vi "GetWindowICCProfile.vi"(8 "No Error":errorcluster, 11 "Window [SDL_Window *]":i64 format="%.0x") -> (0 "Error Out":errorcluster, 3 "ICC Profile Data":u8[](array[numeric]))   [LabVIEW 2026, in "SDL3.lvlib" / "Video.lvlib"]
doc: "<B>Summary</B>\nGet the raw ICC profile data for the screen the window is currently on."
uses:
  Video.lvlib
  <vilib>/Utility/error.llb/Error Cluster From Error Code.vi
  Stdinc/Stdinc.lvlib
  Error/Error.lvlib
  Lib/SDL3.dll
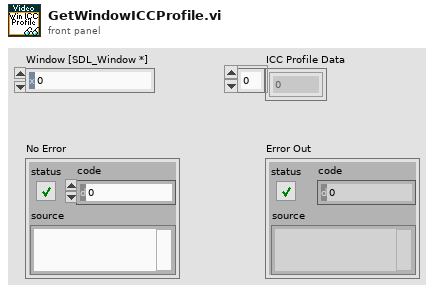
[diagram p1: front panel]
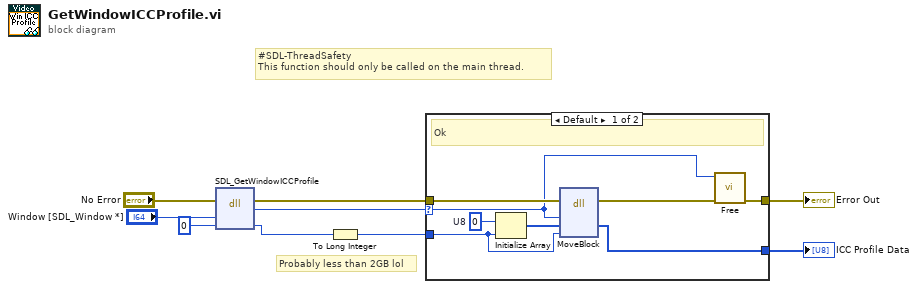
[diagram p0: block diagram]
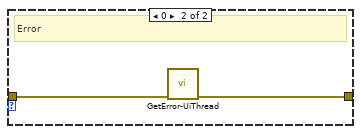
[diagram p2: hidden frame]
diagram:
  # "#SDL-ThreadSafety\nThis function should only be called on the main thread."
  # "Probably less than 2GB lol"
  n1 = dll-call lib="C:/Users/saukko/Dev/LV-SDL3/Sources/SDL3/Lib/SDL3.*" fn="SDL_GetWindowICCProfile"(error in="No Error", "window"="Window [SDL_Window *]", "size"=u64 0) -> (error out=w7:errorcluster, "return type"=w6:i64, "size"=w5:u64)  [unwired: 3 in, 1 out]
  n2 = To Long Integer(number=w5) -> (32bit integer=w2:i32)
  n3 = case shown="Default" w6 {
    selector: w6 -> [w12 _]
    tunnel: w7 -> [w17 w19]
    tunnel: [w13 w18] -> w8
    tunnel: w2 -> [w10 _]
    tunnel: [w14 _] -> w1
    frame Default {
      w11 = u8 0  # U8
      # "Ok"
      n4 = Initialize Array(w11, w10) -> (w15:u8[])
      n5 = dll-call lib="LabVIEW" fn="MoveBlock"(error in=w17, "Address"=w12, "Destination"=w15, "Size"=w10) -> (error out=w16:errorcluster, "Destination"=w14:u8[])  [unwired: 5 in, 1 out]
      n6 = call "Free.vi"("No Error"=w16, "Mem [void *]"=w12) -> ("Error Out"=w13:errorcluster)  [unwired: 9 in]
    }
    frame 0 {
      # "Error"
      n7 = call "GetError-UiThread.vi"("No Error"=w19) -> ("error out"=w18:errorcluster)  [unwired: 10 in]
    }
  }
  "Error Out" <- w8
  "ICC Profile Data" <- w1
